vi "programa 6 archivos cluster.vi"() -> ()   [LabVIEW 2011]
panel:
  out "Array":T1(array[cluster]) {"velocidad 3" scale=0.0..180.0; "velocidad 2" scale=0.0..180.0; "velocidad" scale=0.0..180.0}
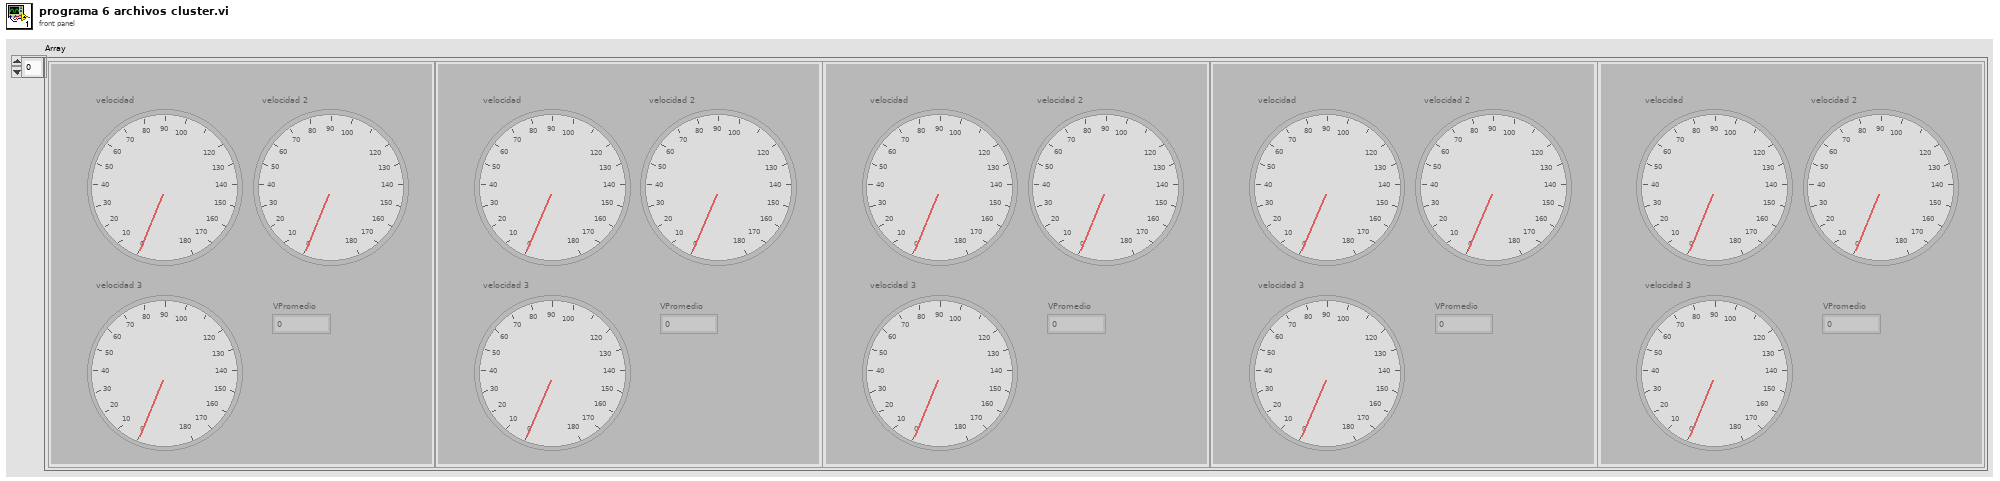
[diagram p1: front panel]
types:
  T1 = cluster{"velocidad":i32, "velocidad 2":i32, "velocidad 3":i32, "VPromedio":dbl}[]
  T2 = enum16{"open", "replace", "create", "open or create", "replace or create", "replace or create with confirmation"}
  T3 = cluster{"velocidad":i32, "velocidad 2":i32, "velocidad 3":i32, "VPromedio":dbl}
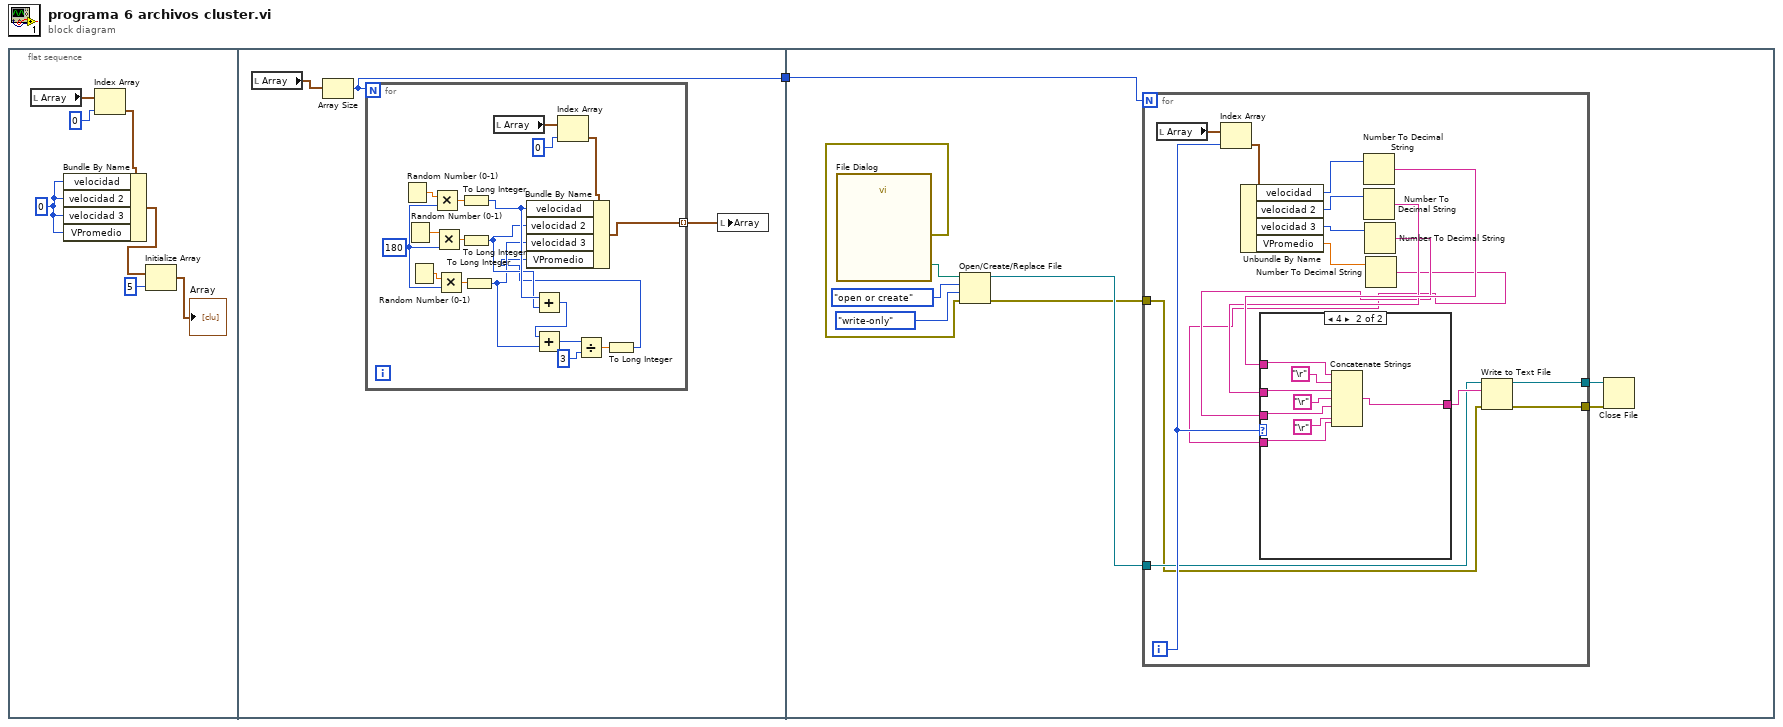
[diagram p0: block diagram]
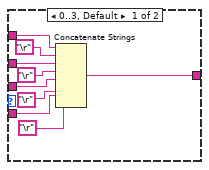
[diagram p2: hidden frame]
diagram:
  n1 = flat-sequence {
    tunnel: [w9] -> w1
    tunnel: w1 -> [w39]
    frame #0 {
      w5 = 0
      n2 = local read "Array"() -> (w8:T1)
      n3 = Index Array "Index Array"(array=w8, index=0) -> (element=w6:T3)
      n4 = Bundle By Name "Bundle By Name"(cluster=w6, "velocidad"=w5, "velocidad 2"=w5, "velocidad 3"=w5, "VPromedio"=w5) -> (w4:T3)
      n5 = Initialize Array "Initialize Array"(w4, 5 ("dimension size")) -> (→"Array":T1)
    }
    frame #1 {
      n6 = local read "Array"() -> (w11:T1)
      n7 = Array Size(array=w11) -> (size(s)=w9:i32)
      n8 = for {
        N: w9 -> [_]
        tunnel: [w12] -> w10 mode=indexing
        w30 = 180
        n9 = Random Number (0-1)() -> (number: 0 to 1=w29:dbl)
        n10 = Random Number (0-1)() -> (number: 0 to 1=w28:dbl)
        n11 = Random Number (0-1)() -> (number: 0 to 1=w27:dbl)
        n12 = Multiply(x=w29, y=w30) -> (x*y=w26:dbl)
        n13 = Multiply(x=w28, y=w30) -> (x*y=w25:dbl)
        n14 = Multiply(x=w27, y=w30) -> (x*y=w24:dbl)
        n15 = To Long Integer(number=w26) -> (32bit integer=w20:i32)
        n16 = To Long Integer(number=w25) -> (32bit integer=w19:i32)
        n17 = To Long Integer(number=w24) -> (32bit integer=w17:i32)
        n18 = local read "Array"() -> (w21:T1)
        n19 = Add(x=w20, y=w19) -> (x+y=w18:i32)
        n20 = Add(x=w18, y=w17) -> (x+y=w16:i32)
        n21 = Index Array "Index Array"(array=w21, index=0) -> (element=w23:T3)
        n22 = Divide(x=w16, y=3) -> (x/y=w14:dbl)
        n23 = To Long Integer(number=w14) -> (32bit integer=w13:i32)
        n24 = Bundle By Name "Bundle By Name"(cluster=w23, "velocidad"=w20, "velocidad 2"=w19, "velocidad 3"=w17, "VPromedio"=w13) -> (w12:T3)
      }
      n25 = local write "Array"(w10) -> ()
    }
    frame #2 {
      n26 = call "File Dialog"() -> ("selected path"=w37:path, "error out"=w38:errorcluster)  [unwired: 12 in, 2 out]
      n27 = Open/Create/Replace File(file path (use dialog)=w37, error in=w38, operation (0:open)=T2."open or create", access (0:read/write)=enum16{"read/write", "read-only", "write-only"}."write-only") -> (refnum out=w34:refnum<file>, error out=w33:errorcluster)  [unwired: 2 in, 1 out]
      n28 = for {
        N: w39 -> [_]
        tunnel: w34 -> [w43]
        tunnel: w33 -> [w42]
        tunnel: [w41] -> w32
        tunnel: [w40] -> w31
        i -> [w49]
        n29 = local read "Array"() -> (w55:T1)
        n30 = Index Array "Index Array"(array=w55, index=w49) -> (element=w54:T3)
        n31 = Unbundle By Name "Unbundle By Name"(w54) -> ("velocidad"=w53:i32, "velocidad 2"=w52:i32, "velocidad 3"=w51:i32, "VPromedio"=w50:dbl)
        n32 = Number To Decimal String(number=w53) -> (decimal integer string=w48:string)  [unwired: 1 in]
        n33 = Number To Decimal String(number=w52) -> (decimal integer string=w47:string)  [unwired: 1 in]
        n34 = Number To Decimal String(number=w51) -> (decimal integer string=w46:string)  [unwired: 1 in]
        n35 = Number To Decimal String(number=w50) -> (decimal integer string=w45:string)  [unwired: 1 in]
        n36 = case shown="4" w49 {
          tunnel: w48 -> [w64 w69]
          tunnel: w47 -> [w62 w68]
          tunnel: w46 -> [w60 w67]
          tunnel: w45 -> [w58 w66]
          tunnel: [w56 w65] -> w44
          frame 0..3, Default {
            n37 = Concatenate Strings "Concatenate Strings"(w64, "\r", w62, "\r", w60, "\r", w58, "\r") -> (w56:string)
          }
          frame 4 {
            n38 = Concatenate Strings "Concatenate Strings"(w69, "\r", w68, "\r", w67, "\r", w66) -> (w65:string)
          }
        }
        n39 = Write to Text File(file (use dialog)=w43, text=w44, error in=w42) -> (refnum out=w41:refnum<file>, error out=w40:errorcluster)  [unwired: 1 in, 1 out]
      }
      n40 = Close File(refnum=w32, error in=w31) -> ()  [unwired: 2 out]
    }
  }
